vi "Calculate P_alt, rho_alt, rho, dew_pt.vi"(0 "Temperature (degC)":sgl, 1 "Pressure (Pa)":sgl, 2 "Rel. Hum. (%)":sgl) -> (3 "Density (kg/m^3)":sgl, 4 "Dew point (degC)":sgl, 5 "Pressure alt. (m)":sgl, 6 "Density alt. (m)":sgl)   [LabVIEW 2015]
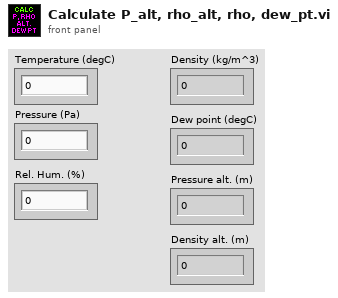
[diagram p1: front panel]
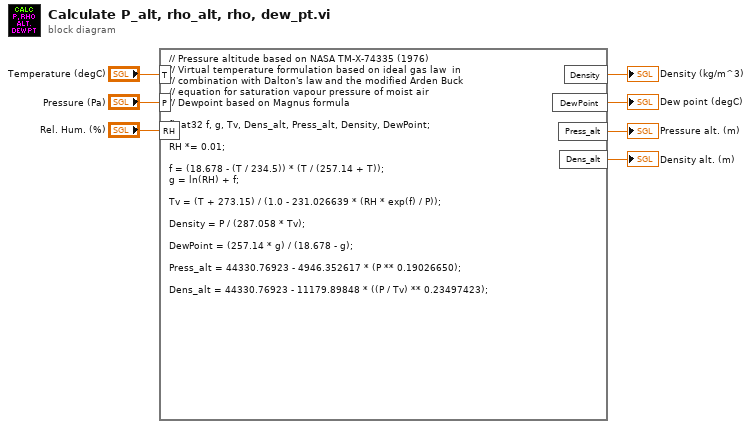
[diagram p0: block diagram]
diagram:
  n1 = formula code="// Pressure altitude based on NASA TM-X-74335 (1976)\n// Virtual temperature formulation based on ideal gas law  in\n// combination with Dalton's law and the modified Arden Buck\n// equation for saturation vapour pressure of moist air\n// Dewpoint based on Magnus formula\n\nfloat32 f, g, Tv, Dens_alt, Press_alt, Density, DewPoint;\n\nRH *= 0.01;\n\nf = (18.678 - (T / 234.5)) * (T / (257.14 + T));\ng = ln(RH) + f;\n\nTv = (T + 273.15) / (1.0 - 231.026639 * (RH * exp(f) / P));\n\nDensity = P / (287.058 * Tv);\n\nDewPoint = (257.14 * g) / (18.678 - g);\n\nPress_alt = 44330.76923 - 4946.352617 * (P ** 0.19026650);\n\nDens_alt = 44330.76923 - 11179.89848 * ((P / Tv) ** 0.23497423);"("P"="Pressure (Pa)", "T"="Temperature (degC)", "RH"="Rel. Hum. (%)") -> ("Dens_alt"=→"Density alt. (m)":sgl, "Press_alt"=→"Pressure alt. (m)":sgl, "Density"=→"Density (kg/m^3)":sgl, "DewPoint"=→"Dew point (degC)":sgl)
